vi "data_y_setGet.vi"(0 "XY":sgl[][](array[numeric]) format="%.2f", 3 "Y":sgl[](array[numeric]) format="%.2f", 9 "mode":enum16{"get", "set"}(ring)) -> (14 "XY out":sgl[][](array[numeric]) format="%.2f", 17 "Y out":sgl[](array[numeric]) format="%.2f")   [LabVIEW 2010]
doc: "SubVI to a <B>Thorlabs_OSA_64</B> object.\n\n[GOOP 1.0]"
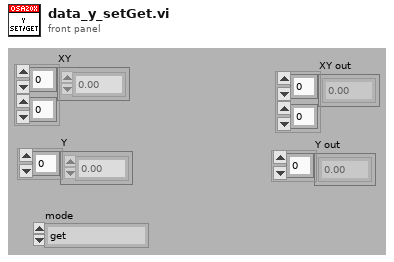
[diagram p1: front panel]
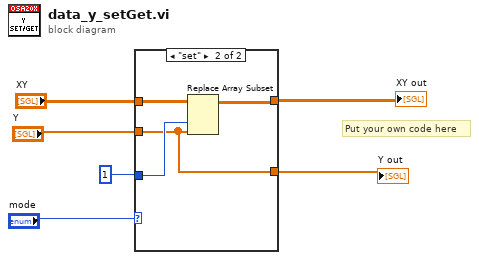
[diagram p0: block diagram]
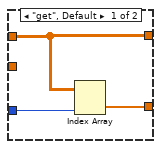
[diagram p2: hidden frame]
diagram:
  # "Put your own code here"
  n1 = case shown="\"set\"" "mode" {
    tunnel: "XY" -> [w8 w13]
    tunnel: [w9 w10] -> w5
    tunnel: [w8 w12] -> w3
    tunnel: 1 ("disabled index (col)") -> [w7 w11]
    tunnel: "Y" -> [_ w10]
    frame "get", Default {
      n2 = Index Array(array=w8, index (col)=w7) -> (element=w9:sgl[])  [unwired: 1 in]
    }
    frame "set" {
      n3 = Replace Array Subset(array=w13, new element=w10, index (col)=w11) -> (w12:sgl[][])  [unwired: 1 in]
    }
  }
  "Y out" <- w5
  "XY out" <- w3
